vi "Create Interaction.vi"(8 "error in":errorcluster, 9 "parameters":cluster{"name":string, "type":string}[](array[cluster]), 10 "name":string, 11 "Item Ref in":T1 format="%.0x") -> (0 "error out":errorcluster, 3 "Item Ref out":T1 format="%.0x")   [LabVIEW 2019, in "HLA Custom Device System Explorer.lvlib"]
uses:
  HLA Custom Device System Explorer.lvlib
  <vilib>/NI VeriStand/Custom Device API/Custom Device Item Ref.ctl
  Shared/Constants.vi
  <vilib>/NI VeriStand/Custom Device API/Custom Device API.lvlib
  Shared/HLA Custom Device Shared.lvlib
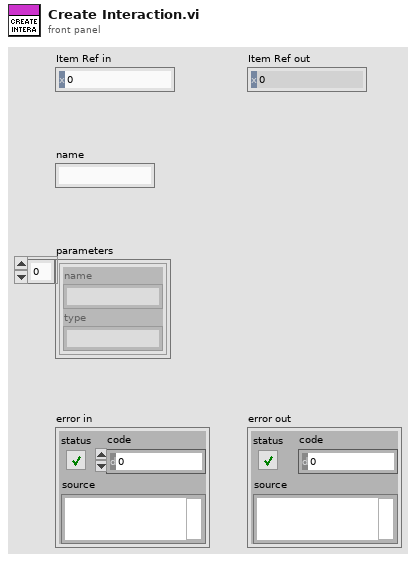
[diagram p1: front panel]
types:
  T1 = typedef "Custom Device API.lvlib/Custom Device Item Ref.ctl" = u64
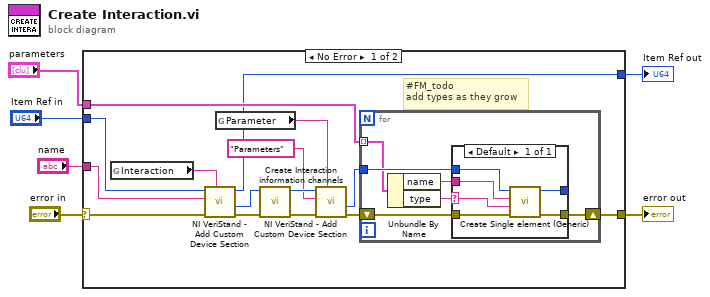
[diagram p0: block diagram]
diagram:
  n1 = case shown="No Error" "error in" {
    selector: "error in" -> [w7 w34]
    tunnel: [w12 w34] -> w6
    tunnel: "parameters" -> [w11 _]
    tunnel: "name" -> [w10 _]
    tunnel: "Item Ref in" -> [w9 w35]
    tunnel: [w8 w35] -> w2
    frame No Error {
      # "#FM_todo\nadd types as they grow"
      n2 = global read "Constants.vi" "Interaction"() -> (w21:string)
      n3 = call <vilib>:"NI VeriStand - Add Custom Device Section.vi"("GUID (Default Section)"=w21, "error in (no error)"=w7, "Section Name"=w10, "Parent Ref in"=w9) -> ("error out"=w14:errorcluster, "Section Ptr"=w13:T1, "Parent Ref out"=w8:T1)  [unwired: 4 in, 1 out]
      n4 = global read "Constants.vi" "Parameter"() -> (w20:string)
      n5 = call "Create Interaction information channels.vi"("error in"=w14, "Item Ref in"=w13) -> ("error out"=w16:errorcluster, "Item Ref out"=w17:T1)  [unwired: 8 in]
      n6 = call <vilib>:"NI VeriStand - Add Custom Device Section.vi"("GUID (Default Section)"=w20, "error in (no error)"=w16, "Section Name"="Parameters", "Parent Ref in"=w17) -> ("error out"=w19:errorcluster, "Section Ptr"=w18:T1)  [unwired: 4 in, 2 out]
      n7 = for {
        shift-right: [w24] -> w12
        shift-left: w19 -> [w27]
        tunnel: w11 -> [w23] mode=indexing
        tunnel: w18 -> [w26]
        n8 = Unbundle By Name(w23) -> ("name"=w25:string, "type"=w22:string)
        n9 = case shown="Default" w22 {
          selector: w22 -> [w31]
          tunnel: w27 -> [w32]
          tunnel: w26 -> [w33]
          tunnel: w25 -> [w28]
          tunnel: [w30] -> _
          tunnel: [w29] -> w24
          frame Default {
            n10 = call "Create Single element (Generic).vi"("error in"=w32, "type"=w31, "name"=w28, "Item Ref in"=w33) -> ("error out"=w29:errorcluster, "Item Ref out"=w30:T1)  [unwired: 6 in]
          }
        }
      }
    }
    frame Error {
    }
  }
  "Item Ref out" <- w2
  "error out" <- w6
